vi "Write_Config.vi"() -> ()   [LabVIEW 2025]
uses:
  D:/LV test/LabVIEWConfigSecurity.dll
  LabVIEWConfigSecurity.dll
panel:
  in  "簇":cluster{"Speed":dbl, "MachineName":string}={"Speed"=1500.0, "MachineName"="liq_z"}
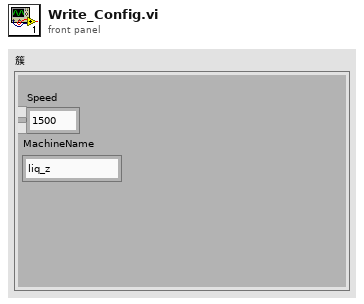
[diagram p1: front panel]
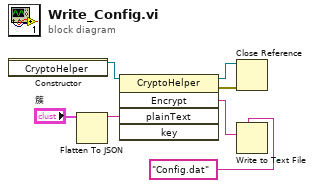
[diagram p0: block diagram]
diagram:
  n1 = constructor class="CryptoHelper"() -> (reference out=w6:refnum<k24>)  [unwired: 3 in, 2 out]
  n2 = Flatten To JSON(anything="簇") -> (JSON string=w5:string)  [unwired: 2 in, 1 out]
  n3 = invoke on="调用节点" class="CryptoHelper" method="Encrypt"(reference=w6, "plainText"=w5) -> (reference out=w1:refnum<k24>, error out=w2:errorcluster, "Encrypt"=w3:string)  [unwired: 3 in, 2 out]
  n4 = Close Reference(reference=w1, error in (no error)=w2) -> ()  [unwired: 1 out]
  n5 = Write to Text File(prompt (Choose or enter file path)="Config.dat", text=w3) -> ()  [unwired: 2 in, 3 out]
